vi "CSM-Logger-Thread(Event).vi"(4 "Log Limit":T1={"file size (in bytes)"=10000000, "file num"=2} {"file size (in bytes)" format="%.0p"}, 6 "Exit When All Module Exist? (F)":bool, 7 "Format String":string="%<%Y/%m/%d %H:%M:%S%3u>T", 8 "error in (no error)":errorcluster, 9 "WatchDogQ":refnum<queue>, 10 "GlobalLogFilter.lvclass":refnum<class "LogFilter.lvclass">, 11 "File Path (Use Dialog)":path) -> (0 "error out":errorcluster)   [LabVIEW 2017, in "CSM File Logger.lvlib"]
uses:
  CSM File Logger.lvlib
  CSM File Logger Limit.ctl
  _Support/GlobalEvent/LogFilter/LogFilter.lvclass
  _Support/Typedef/_CSM_List Module Scope.ctl
  _Support/Typedef/_CSM_GlobalLog_MSG.ctl
  _Support/Typedef/_CSM_Response Source Message.ctl
  _Support/Typedef/_CSM_GlobalLog_MSG_TYPE.ctl
  Utility/_support/Periodic String Filter Level.ctl
  _Support/GlobalEvent/GEvt-Generate with Rule Check.vi
  AdvanceAPI/CSM - Convert Error to Argument.vi
  AdvanceAPI/CSM - Make String Arguments Safe.vi
  AdvanceAPI/CSM - Keywords.vi
  _Support/GlobalEvent/Cache-GEvt Refs.vi
  Communicable State Machine.lvlib
panel:
  out "size (in bytes)":i64
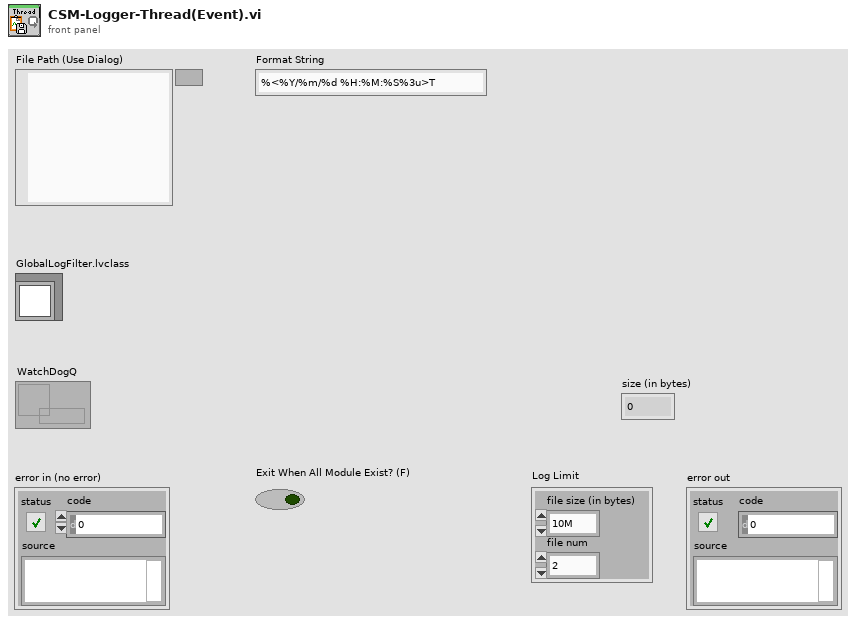
[diagram p1: front panel]
types:
  T1 = typedef "CSM File Logger.lvlib/CSM File Logger Limit.ctl" = cluster{"file size (in bytes)":i64, "file num":i32}
  T2 = typedef "Communicable State Machine.lvlib/_CSM_GlobalLog_MSG_TYPE.ctl" = enum16{"User Log", "State Change", "Status", "Interrupt", "Register", "Unregister", "Error Log", "Module Created", "Module Destroyed"}
  T3 = typedef "Communicable State Machine.lvlib/_CSM_GlobalLog_STATE_TYPE.ctl" = enum16{"State - Internal State", "State - External Message", "State - Response", "State - Complete"}
  T4 = cluster{"Global":cluster{"CSM":string[], "LogType":T2[], "State":string[], "StateType":T3[]}, "CSM":cluster{"LogType":cluster{"CSM":string, "LogType":T2}[], "State":cluster{"CSM":string, "State":string}[], "StateType":cluster{"CSM":string, "LogType":T3}[]}, "PeriodicLog":cluster{"Enable":bool, "Threshold(#/s)":dbl, "CheckPeriod(s)":dbl}}
  T5 = cluster{"Queue":path[], "folder":path, "name":string, "index":i32, "Log Limit":T1}
  T6 = typedef "Communicable State Machine.lvlib/_CSM_List Module Scope.ctl" = enum16{"Normal", "System Only", "All"}
  T7 = typedef "Communicable State Machine.lvlib/Periodic String Filter Level.ctl" = enum16{"normal", "L1", "L2", "L3", "L4"}
  T8 = typedef "Communicable State Machine.lvlib/_CSM_GlobalLog_MSG.ctl" = cluster{"Name (\"\" to Use UUID)":string, "Current State":string, "Arguments":string, "Source Message":T9, "Source Module":string, "Complete(T)/Start(F)":bool, "LogType":T2, "Time Stamp":timestamp}
  T9 = typedef "Communicable State Machine.lvlib/_CSM_Response Source Message.ctl" = cluster{"‘State":string, "’Arguments":string, "’Error":errorcluster}
  T10 = enum16{"open", "replace", "create", "open or create", "replace or create", "replace or create with confirmation"}
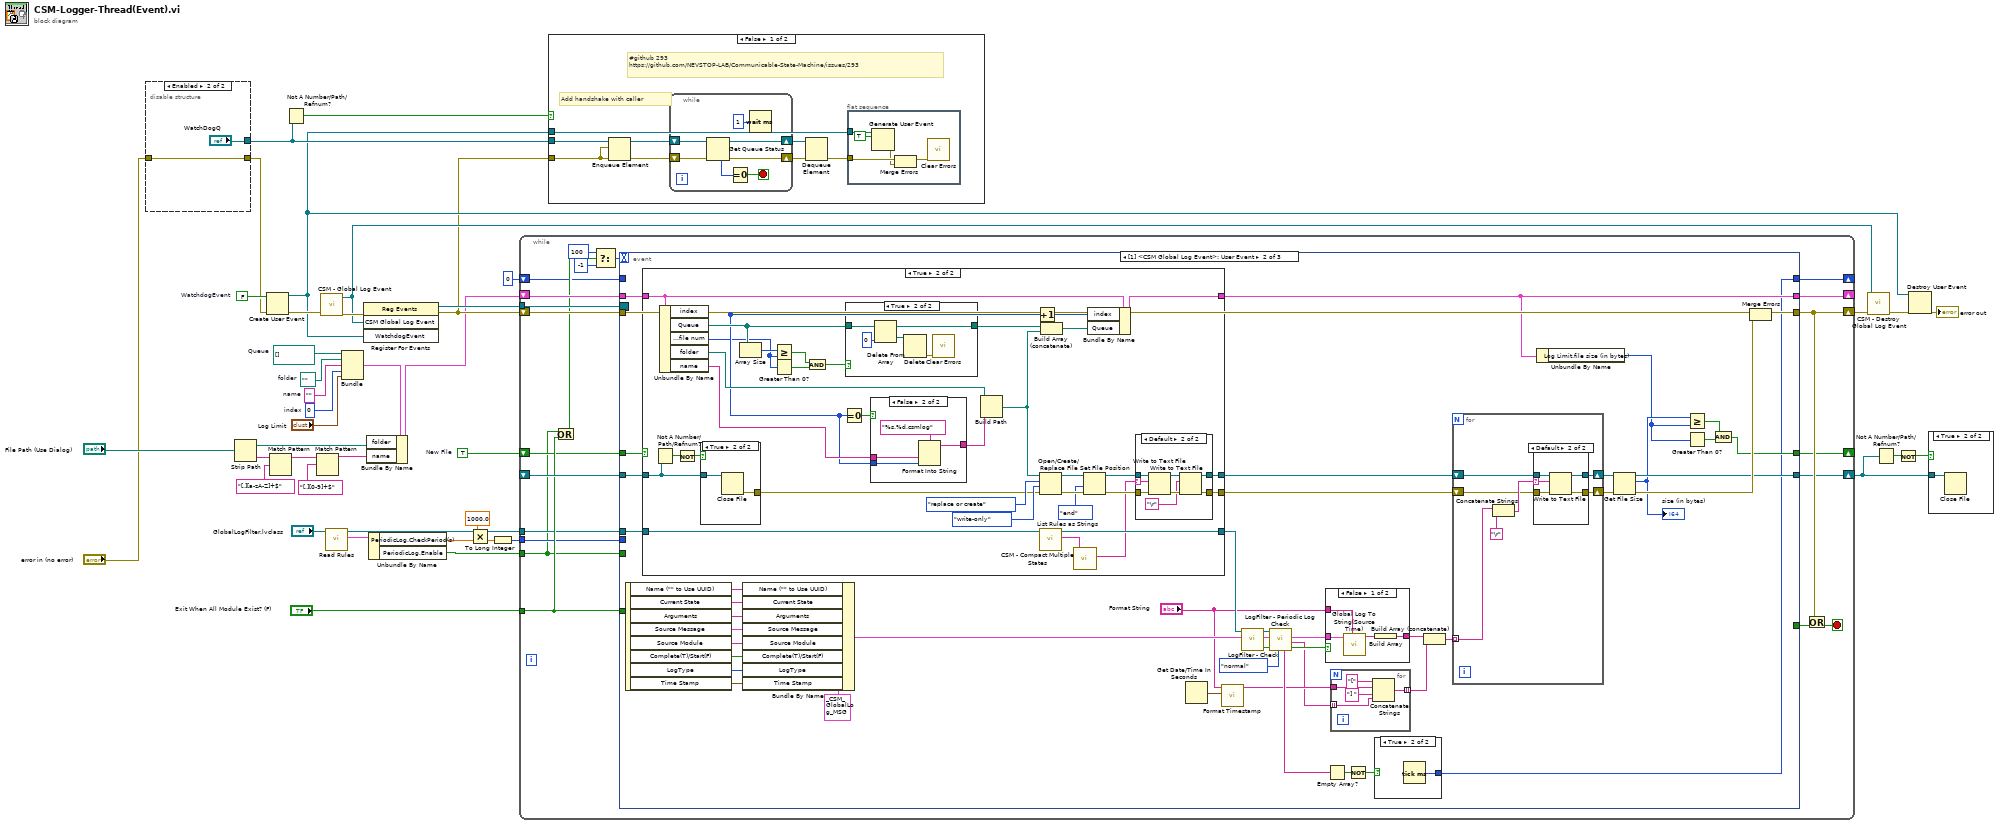
[diagram p0: block diagram]
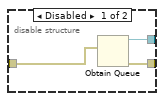
[diagram p2: hidden frame]
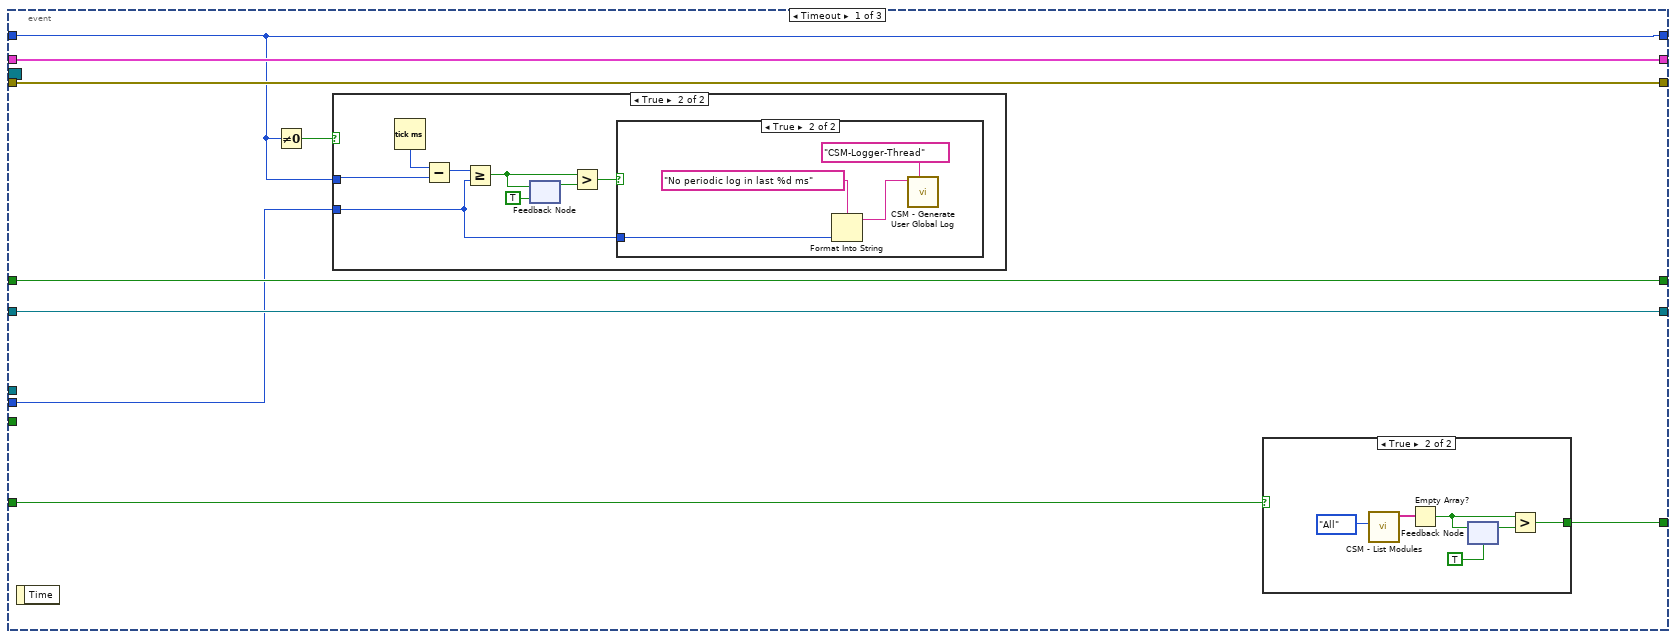
[diagram p5: hidden frame]
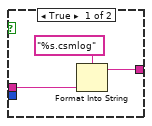
[diagram p14: hidden frame]
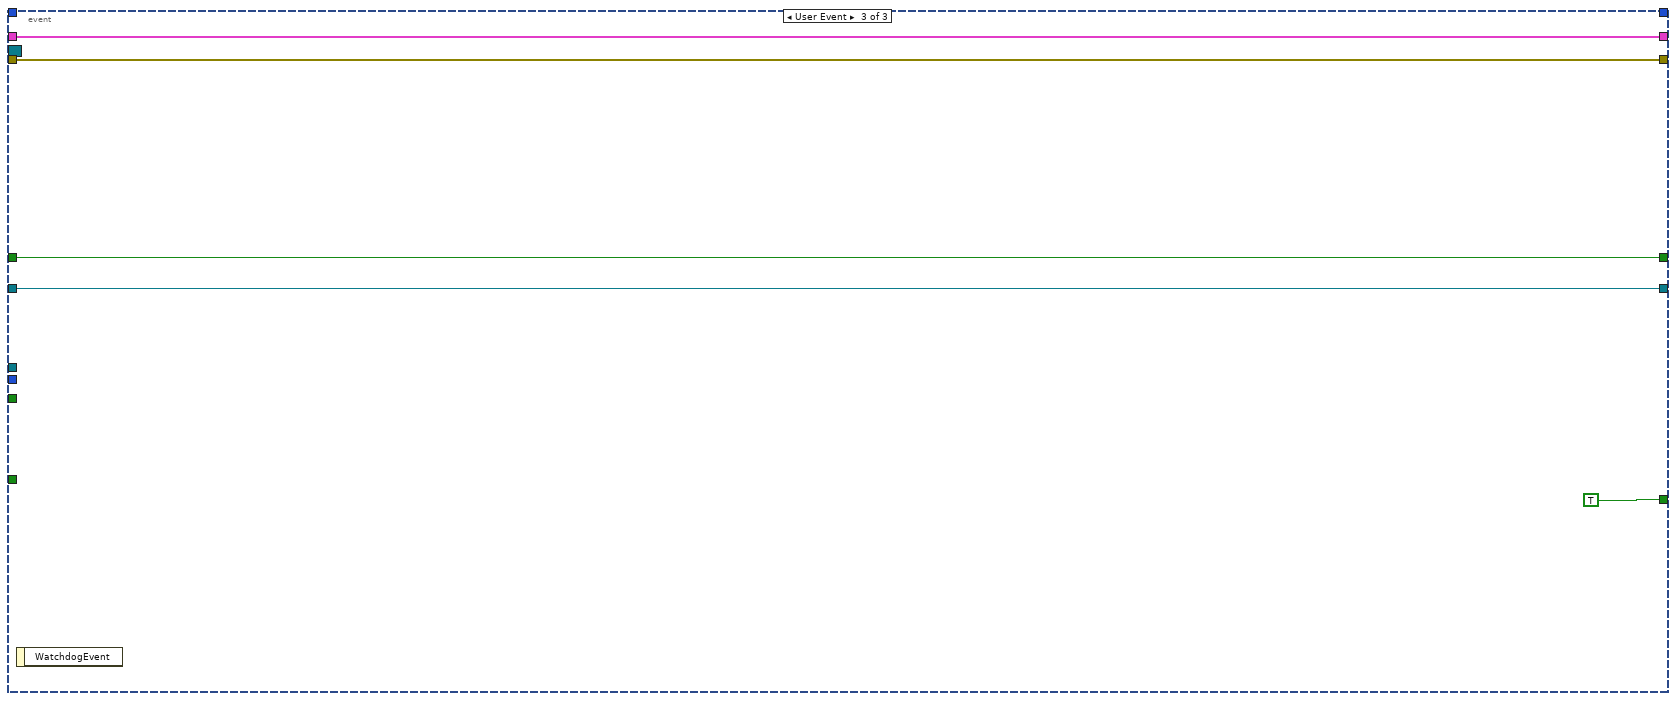
[diagram p17: hidden frame]
diagram:
  w19 = ""  # name
  w22 = 0  # index
  w23 = path ""  # folder
  w24 = path[] []  # Queue
  w27 = TRUE  # New File
  w36 = FALSE  # WatchdogEvent
  n1 = disable-structure shown="Enabled" {
    disable-tunnel: [w43 "WatchDogQ"] -> w38
    disable-tunnel: [w45 w46] -> w26
    disable-tunnel: "error in (no error)" -> [w44 w46]
    frame Disabled {
      n2 = Obtain Queue(element data type=w44) -> (queue out=w43:refnum<queue>, error out=w45:errorcluster)  [unwired: 4 in, 1 out]
    }
    frame Enabled {
    }
  }
  n3 = Strip Path(path="File Path (Use Dialog)") -> (stripped path=w12:path, name=w18:string)
  n4 = Create User Event(user event datatype=w36, error in=w26) -> (user event=w33:refnum<user-event>, error out=w35:errorcluster)
  n5 = Match Pattern(string=w18, regular expression="[.][a-zA-Z]+$") -> (before substring=w15:string)  [unwired: 1 in, 3 out]
  n6 = Not A Number/Path/Refnum?(number/path/refnum=w38) -> (NaN/Path/Refnum?=w37:bool)
  n7 = Match Pattern(string=w15, regular expression="[.][0-9]+$") -> (before substring=w13:string)  [unwired: 1 in, 3 out]
  n8 = call "CSM - Global Log Event.vi"("Error In"=w35) -> ("error out"=w40:errorcluster, "CSM Global Log Event"=w39:refnum<user-event>)  [unwired: 9 in]
  n9 = call "Read Rules.vi"("LogFilter In"="GlobalLogFilter.lvclass") -> ("Rules"=w7:T4, "LogFilter Out"=w8:refnum<class "LogFilter.lvclass">)  [unwired: 8 in, 1 out]
  n10 = Bundle("Queue"=w24, "folder"=w23, "name"=w19, "index"=w22, "Log Limit"="Log Limit") -> (w20:T5)  [unwired: 1 in]
  n11 = register-events(error in=w40, w39, w33) -> (reference out=w42:refnum<event-registration>, error out=w25:errorcluster)  [unwired: 1 in]
  n12 = Bundle By Name(cluster=w20, "folder"=w12, "name"=w13) -> (w14:T5)
  n13 = Unbundle By Name(w7) -> ("PeriodicLog.CheckPeriod(s)"=w5:dbl, "PeriodicLog.Enable"=w6:bool)
  n14 = Multiply(x=1000.0, y=w5) -> (x*y=w4:dbl)
  n15 = To Long Integer(number=w4) -> (32bit integer=w2:i32)
  n16 = while {
    tunnel: w42 -> [w68]
    shift-right: [w65] -> w41
    shift-left: w25 -> [w67]
    shift-right: [w62] -> w30
    shift-left: _ -> [w63]
    tunnel: "Exit When All Module Exist? (F)" -> [w61]
    shift-right: [w57] -> _
    shift-left: w27 -> [w58]
    shift-right: [w55] -> _
    shift-left: w14 -> [w56]
    tunnel: w8 -> [w54]
    tunnel: w6 -> [w49]
    tunnel: w2 -> [w53]
    shift-right: [w52] -> _
    shift-left: u32 0 ("millisecond timer value") -> [w48]
    stop <- w66 stop-if-true
    n17 = Or(x=w49, y=w61) -> (x .or. y?=w50:bool)
    n18 = Select(t=100, s=w50, f=-1) -> (s? t:f=w59:i32)
    n19 = event shown="[1] <CSM Global Log Event>: User Event" {
      selector: w68 -> [_ _ _]
      dyn-events: _ -> [_ _ _]
      timeout: w59 -> [_ _ _]
      tunnel: w67 -> [w77 w132 w232]
      tunnel: [w77 w131 w232] -> w65
      tunnel: [w75 _ TRUE ("rising edge")] -> w64
      tunnel: w63 -> [w76 w133 w231]
      tunnel: [w76 w124 w231] -> w62
      tunnel: w61 -> [w74 _ _]
      tunnel: w58 -> [w73 w128 w229]
      tunnel: [w73 w122 w229] -> w57
      tunnel: w56 -> [w72 w117 w228]
      tunnel: [w72 w118 w228] -> w55
      tunnel: w54 -> [_ w114 _]
      tunnel: w49 -> [_ _ _]
      tunnel: w53 -> [w69 _ _]
      tunnel: [w70 w102 _] -> w52
      tunnel: w48 -> [w70 _ _]
      event Timeout {
        n20 = event-data() -> ()  [unwired: 1 in, 1 out]
        n21 = Not Equal To 0?(x=w70) -> (x != 0?=w71:bool)
        n22 = case shown="True" w71 {
          tunnel: w70 -> [_ w84]
          tunnel: w69 -> [_ w79]
          frame False {
          }
          frame True {
            n23 = Tick Count (ms)() -> (millisecond timer value=w85:u32)
            n24 = Subtract(x=w85, y=w84) -> (x-y=w83:u32)
            n25 = Greater Or Equal?(x=w83, y=w79) -> (x >= y?=w82:bool)
            n26 = feedback-in #1(w82) -> ()
            n27 = feedback #1(TRUE) -> (w81:bool)
            n28 = Greater?(x=w82, y=w81) -> (0:w78:bool)
            n29 = case shown="True" w78 {
              tunnel: w79 -> [_ w86]
              frame False {
              }
              frame True {
                n30 = Format Into String(format string="No periodic log in last %d ms" ("Log"), w86) -> (resulting string=w87:string)  [unwired: 2 in, 1 out]
                n31 = call "CSM - Generate User Global Log.vi"("Place (\"\" to Use VI's Name)"="CSM-Logger-Thread" ("Place(\"\" to use VI's Name)"), "Log"=w87) -> ()  [unwired: 9 in, 1 out]
              }
            }
          }
        }
        n32 = case shown="True" w74 {
          tunnel: [_ w91] -> w75
          frame False {
          }
          frame True {
            n33 = call "CSM - List Modules.vi"("Scope (Normal)"=_CSM_List_Module_Scope."All" ("Mode")) -> ("Module Names"=w95:string[])  [unwired: 9 in, 1 out]
            n34 = Empty Array?(array=w95) -> (empty?=w94:bool)
            n35 = feedback #2(TRUE ("All?")) -> (w93:bool)
            n36 = feedback-in #2(w94) -> ()
            n37 = Greater?(x=w94, y=w93) -> (0:w91:bool)
          }
        }
      }
      event User Event {
        n38 = event-data() -> ("Name (\"\" to Use UUID)"=w141:string, "Current State"=w140:string, "Arguments"=w139:string, "Source Message"=w138:T9, "Source Module"=w137:string, "Complete(T)/Start(F)"=w136:bool, "LogType"=w135:T2, "Time Stamp"=w101:timestamp)  [unwired: 1 in]
        n39 = case shown="True" w128 {
          tunnel: w133 -> [w168 w200]
          tunnel: [_ w172] -> w130
          tunnel: [w168 w173] -> w129
          tunnel: [w167 w189] -> w118
          tunnel: w117 -> [w167 w191]
          tunnel: [w166 w171] -> w115
          tunnel: w114 -> [w166 w176]
          frame False {
          }
          frame True {
            n40 = Not A Number/Path/Refnum?(number/path/refnum=w200) -> (NaN/Path/Refnum?=w201:bool)
            n41 = Unbundle By Name(w191) -> ("index"=w181:i32, "Queue"=w192:path[], "Log Limit.file num"=w178:i32, "folder"=w185:path, "name"=w184:string)
            n42 = Not(x=w201) -> (.not. x?=w202:bool)
            n43 = case shown="True" w202 {
              tunnel: w200 -> [_ w227]
              tunnel: [_ w226] -> w194
              frame False {
              }
              frame True {
                n44 = Close File(refnum=w227) -> (error out=w226:errorcluster)  [unwired: 1 in, 1 out]
              }
            }
            n45 = Array Size(array=w192) -> (size(s)=w193:i32)
            n46 = Greater Or Equal?(x=w193, y=w178) -> (x >= y?=w180:bool)
            n47 = Greater Than 0?(x=w178) -> (x > 0?=w179:bool)
            n48 = And(x=w180, y=w179) -> (x .and. y?=w177:bool)
            n49 = Equal To 0?(x=w181) -> (x = 0?=w182:bool)
            n50 = case shown="True" w177 {
              tunnel: w192 -> [w220 w225]
              tunnel: [w220 w221] -> w190
              frame False {
              }
              frame True {
                n51 = Delete From Array(array=w225, index=0) -> (deleted portion=w223:path, array with subset deleted=w221:path[])  [unwired: 1 in]
                n52 = Delete(path (use dialog)=w223) -> (error out=w222:errorcluster)  [unwired: 4 in, 2 out]
                n53 = call <vilib>:"Clear Errors.vi"("error in (no error)"=w222) -> ()  [unwired: 5 in, 2 out]
              }
            }
            n54 = case shown="False" w182 {
              tunnel: [w214 w218] -> w186
              tunnel: w184 -> [w213 w217]
              tunnel: w181 -> [_ w216]
              frame True {
                n55 = Format Into String(format string="%s.csmlog", w213) -> (resulting string=w214:string)  [unwired: 2 in, 1 out]
              }
              frame False {
                n56 = Format Into String(format string="%s.%d.csmlog", w217, w216) -> (resulting string=w218:string)  [unwired: 2 in, 1 out]
              }
            }
            n57 = Build Path(base path=w185, name or relative path=w186) -> (appended path=w183:path)
            n58 = Increment(x=w181) -> (x+1=w187:i32)
            n59 = call "List Rules as Strings.vi"("GlobalLogFilter In"=w176) -> ("Rule Strings"=w170:string[], "GlobalLogFilter Out"=w171:refnum<class "LogFilter.lvclass">)  [unwired: 8 in, 1 out]
            n60 = Open/Create/Replace File(file path (use dialog)=w183, error in=w194, operation (0:open)=T10."replace or create", access (0:read/write)=enum16{"read/write", "read-only", "write-only"}."write-only") -> (refnum out=w199:refnum<file>, error out=w198:errorcluster)  [unwired: 2 in, 1 out]
            n61 = Build Array (concatenate)(w190, w183) -> (w188:path[])
            n62 = call "CSM - Compact Multiple States.vi"("Multiple States"=w170) -> ("States"=w169:string)  [unwired: 9 in]
            n63 = Set File Position(refnum=w199, from (0:start)=enum16{"start", "end", "current"}."end", error in=w198) -> (refnum out=w174:refnum<file>, error out=w175:errorcluster)  [unwired: 1 in]
            n64 = Bundle By Name(cluster=w191, "index"=w187, "Queue"=w188) -> (w189:T5)
            n65 = case shown="Default" w169 {
              selector: w169 -> [_ w212]
              tunnel: w175 -> [w203 w211]
              tunnel: w174 -> [w204 w210]
              tunnel: [w204 w207] -> w173
              tunnel: [w203 w206] -> w172
              frame "" {
              }
              frame Default {
                n66 = Write to Text File(file (use dialog)=w210, text=w212, error in=w211) -> (refnum out=w208:refnum<file>, error out=w209:errorcluster)  [unwired: 1 in, 1 out]
                n67 = Write to Text File(file (use dialog)=w208, text="\r", error in=w209) -> (refnum out=w207:refnum<file>, error out=w206:errorcluster)  [unwired: 1 in, 1 out]
              }
            }
          }
        }
        n68 = Bundle By Name(cluster=T8 {"Name (\"\" to Use UUID)"="", "Current State"="", "Arguments"="", "Source Message"={"‘State"="", "’Arguments"="", "’Error"={"status"=FALSE, "code"=0, "source"=""}}, "Source Module"="", "Complete(T)/Start(F)"=FALSE, "LogType"=enum."User Log", "Time Stamp"=timestamp(0 s since 1904-01-01)} ("Cross CSM Data"), "Name (\"\" to Use UUID)"=w141, "Current State"=w140, "Arguments"=w139, "Source Message"=w138, "Source Module"=w137, "Complete(T)/Start(F)"=w136, "LogType"=w135, "Time Stamp"=w101) -> (w116:T8)
        n69 = Get Date/Time In Seconds() -> (seconds since 1Jan1904=w108:timestamp)
        n70 = call "Format Timestamp.vi"("Timestamp"=w108, "Format String"="Format String") -> ("String"=w100:string)  [unwired: 9 in]
        n71 = call "LogFilter - Check.vi"("Cross CSM Data In"=w116, "GlobalLogFilter In"=w115) -> ("Matched? (Dup)"=w110:bool, "Cross CSM Data Out"=w111:T8, "GlobalLogFilter.lvclass (Dup)"=w113:refnum<class "LogFilter.lvclass">)  [unwired: 7 in]
        n72 = call "LogFilter - Periodic Log Check.vi"("Level (Normal)"=Periodic_String_Filter_Level."normal" ("Level(Normal)"), "Matched Previous?"=w110, "Cross CSM Data In"=w111, "GlobalLogFilter In"=w113) -> ("Matched? (Dup)"=w107:bool, "Additional Info"=w99:string[], "Cross CSM Data Out"=w112:T8, "Filtered Status"=w105:string[])  [unwired: 3 in, 1 out]
        n73 = case shown="False" w107 {
          tunnel: w112 -> [w165 _]
          tunnel: [w163 _] -> w109
          tunnel: "Format String" -> [w162 _]
          frame False {
            n74 = call "Global Log To String(Source Time).vi"("Format String"=w162, "Log"=w165) -> ("Log String"=w164:string)  [unwired: 8 in]
            n75 = Build Array(w164) -> (w163:string[])
          }
          frame True {
          }
        }
        n76 = Empty Array?(array=w105) -> (empty?=w104:bool)
        n77 = for {
          tunnel: w100 -> [w144]
          tunnel: w99 -> [w143] mode=indexing
          tunnel: [w142] -> w98 mode=indexing
          n78 = Concatenate Strings("[" ("string"), w144, "] " ("string"), w143) -> (w142:string)
        }
        n79 = Not(x=w104) -> (.not. x?=w103:bool)
        n80 = case shown="True" w103 {
          tunnel: [_ w147] -> w102
          frame False {
          }
          frame True {
            n81 = Tick Count (ms)() -> (millisecond timer value=w147:u32)
          }
        }
        n82 = Build Array (concatenate)(w109, w98) -> (w106:string[])
        n83 = for {
          tunnel: w106 -> [w148] mode=indexing
          shift-right: [w150] -> w126
          shift-left: w130 -> [w153]
          shift-right: [w151] -> w127
          shift-left: w129 -> [w152]
          n84 = Concatenate Strings(w148, "\r") -> (w154:string)
          n85 = case shown="Default" w154 {
            selector: w154 -> [_ w161]
            tunnel: w153 -> [w155 w160]
            tunnel: w152 -> [w156 w159]
            tunnel: [w156 w158] -> w151
            tunnel: [w155 w157] -> w150
            frame "" {
            }
            frame Default {
              n86 = Write to Text File(file (use dialog)=w159, text=w161, error in=w160) -> (refnum out=w158:refnum<file>, error out=w157:errorcluster)  [unwired: 1 in, 1 out]
            }
          }
        }
        n87 = Unbundle By Name(w118) -> ("Log Limit.file size (in bytes)"=w119:i64)
        n88 = Get File Size(file=w127, error in=w126) -> (refnum out=w124:refnum<file>, size (in bytes)=w123:i64, 0:w125:errorcluster)
        "size (in bytes)" <- w123
        n89 = Greater Or Equal?(x=w123, y=w119) -> (x >= y?=w121:bool)
        n90 = Greater Than 0?(x=w119) -> (x > 0?=w120:bool)
        n91 = And(x=w121, y=w120) -> (x .and. y?=w122:bool)
        n92 = Merge Errors(w132, w125) -> (w131:errorcluster)
      }
      event User Event {
        n93 = event-data() -> ()  [unwired: 1 in, 1 out]
      }
    }
    n94 = Or(x=w65, y=w64) -> (x .or. y?=w66:bool)
  }
  n95 = case shown="False" w37 {
    tunnel: w38 -> [w238 _]
    tunnel: w33 -> [w239 _]
    tunnel: w25 -> [w233 _]
    frame False {
      # "#github 293 \nhttps://github.com/NEVSTOP-LAB/Communicable-State-Machine/issues/293"
      # "Add handshake with caller"
      n96 = Enqueue Element(queue=w238, element=w233, error in (no error)=w233) -> (queue out=w237:refnum<queue>, error out=w235:errorcluster)  [unwired: 1 in, 1 out]
      n97 = while {
        shift-right: [w246] -> w236
        shift-left: w237 -> [w247]
        shift-right: [w244] -> w234
        shift-left: w235 -> [w245]
        stop <- w242 stop-if-true
        n98 = Get Queue Status(queue=w247, error in (no error)=w245) -> (queue out=w246:refnum<queue>, error out=w244:errorcluster, # elements in queue=w243:i32)  [unwired: 1 in, 5 out]
        n99 = Equal To 0?(x=w243) -> (x = 0?=w242:bool)
        n100 = Wait (ms)(milliseconds to wait=u32 1) -> ()  [unwired: 1 out]
      }
      n101 = Dequeue Element(queue=w236, error in (no error)=w234) -> (error out=w240:errorcluster)  [unwired: 1 in, 3 out]
      n102 = flat-sequence {
        tunnel: w240 -> [w251]
        tunnel: w239 -> [w252]
        frame #0 {
          n103 = Generate User Event(user event=w252, event data cluster=TRUE ("event data")) -> (error out=w249:errorcluster)  [unwired: 2 in, 1 out]
          n104 = Merge Errors(w251, w249) -> (w250:errorcluster)
          n105 = call <vilib>:"Clear Errors.vi"("error in (no error)"=w250) -> ()  [unwired: 5 in, 2 out]
        }
      }
    }
    frame True {
    }
  }
  n106 = call "CSM - Destroy Global Log Event.vi"("Error In"=w41, "CSM Global Log Event"=w39) -> ("error out"=w34:errorcluster)  [unwired: 9 in]
  n107 = Not A Number/Path/Refnum?(number/path/refnum=w30) -> (NaN/Path/Refnum?=w31:bool)
  n108 = Not(x=w31) -> (.not. x?=w29:bool)
  n109 = Destroy User Event(user event=w33, error in=w34) -> (error out=→"error out":errorcluster)
  n110 = case shown="True" w29 {
    tunnel: w30 -> [_ w253]
    frame False {
    }
    frame True {
      n111 = Close File(refnum=w253) -> ()  [unwired: 1 in, 2 out]
    }
  }
